vi "APTset.vi"(7 "Set position":sgl min=0 max=500, 8 "error in (no error)":errorcluster, 11 "reference":refnum<k7>) -> (0 "error out":errorcluster, 3 "reference out":refnum<k7>)   [LabVIEW 2013]
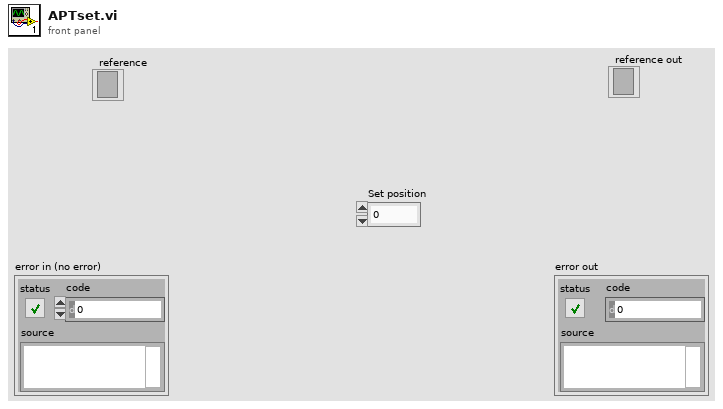
[diagram p1: front panel]
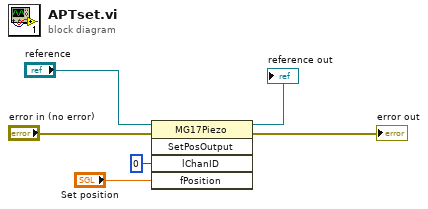
[diagram p0: block diagram]
diagram:
  n1 = invoke class="MG17Piezo" method="SetPosOutput"(reference="reference", error in="error in (no error)", "lChanID"=0, "fPosition"="Set position") -> (reference out=→"reference out":refnum<k7>, error out=→"error out":errorcluster)  [unwired: 1 in, 3 out]
